vi "dmc.vi"() -> ()   [LabVIEW 2016]
panel:
  in  "Customizable Tab":enum32{"Page 1", "Page 2"}(tab)
  in  "Preferences Button":bool
  in  "Start Button":bool
  in  "Boolean Switch":bool
  in  "Horizontal Multi-Slider Control":cluster{"Fill":dbl, "Fill":dbl}(slide)={"Fill"=1.0, "Fill"=8.628318584070797} scale=0.0..200000.0
  in  "Numeric Control":dbl
  in  "Listbox":i32(listbox)
  in  "VISA":refnum<visa-resource-name>
  in  "Radio Buttons - Customizable":T1(radio)
  in  "Enum - Menu":enum16{""}(ring)
  out "Waveform Chart - Dark":dbl(graph) caption="Waveform Chart - dark"
  out "2D Picture":picture
  out "Gauge":dbl(knob) scale=0.0..100000.0
  in  "stop":bool
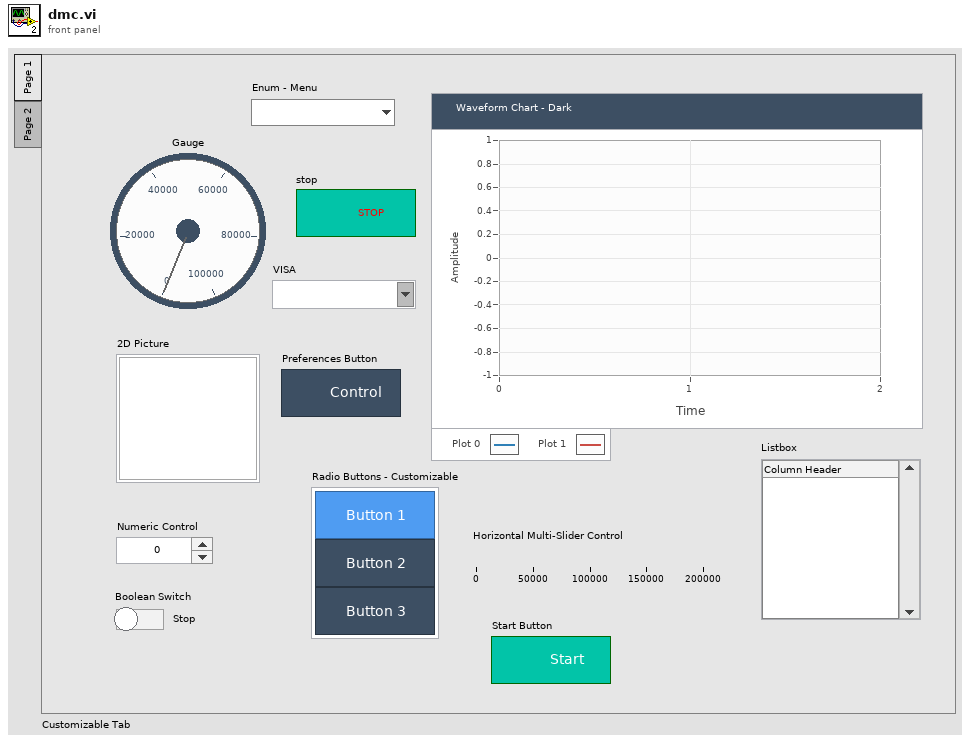
[diagram p1: front panel]
types:
  T1 = enum32{"Standard Button", "Standard Button 2", "Standard Button 3"}
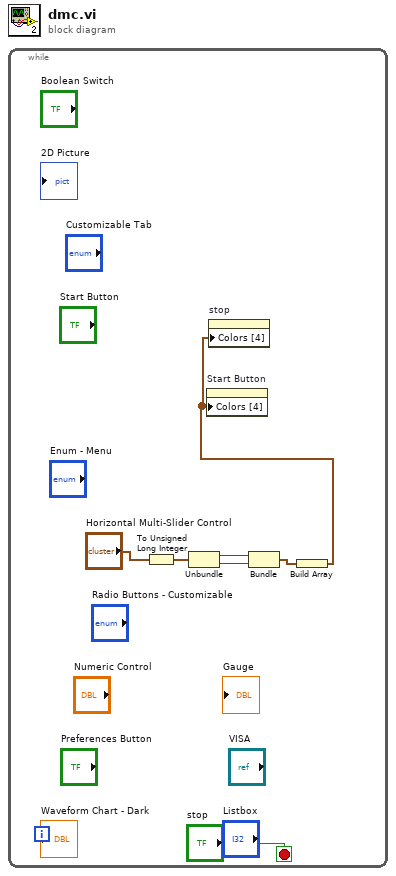
[diagram p0: block diagram]
diagram:
  n1 = while {
    stop <- "stop" stop-if-true
    n2 = To Unsigned Long Integer(number="Horizontal Multi-Slider Control") -> (unsigned 32bit integer=w5:cluster{"Fill":u32, "Fill":u32})
    n3 = Unbundle(w5) -> ("Fill"=w4:u32, "Fill"=w3:u32)
    n4 = Bundle("Fill"=w4, "Fill"=w3) -> (w2:cluster{"Fill":u32, "Fill":u32})  [unwired: 1 in]
    n5 = Build Array(w2) -> (w1:cluster{"Fill":u32, "Fill":u32}[])
    n6 = property on="Start Button" class="Bool"("Colors [4]"=w1) -> ()  [unwired: 2 in, 2 out]
    n7 = property on="stop" class="Bool"("Colors [4]"=w1) -> ()  [unwired: 2 in, 2 out]
  }
